vi "simulate (multiple).vi"(2 "liability?  (benefit)":bool, 3 "estimated values":i16[][](array[numeric]), 4 "source data":i16[](array[numeric])) -> (0 "Array":i16[][](array[numeric]), 1 "correct # of elements in source data?":bool)   [LabVIEW 2009]
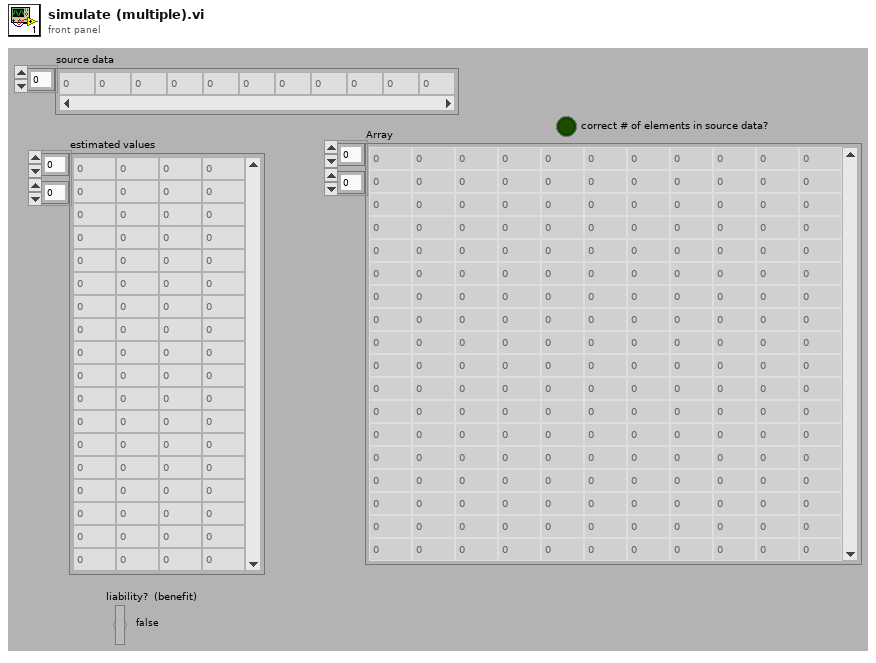
[diagram p1: front panel]
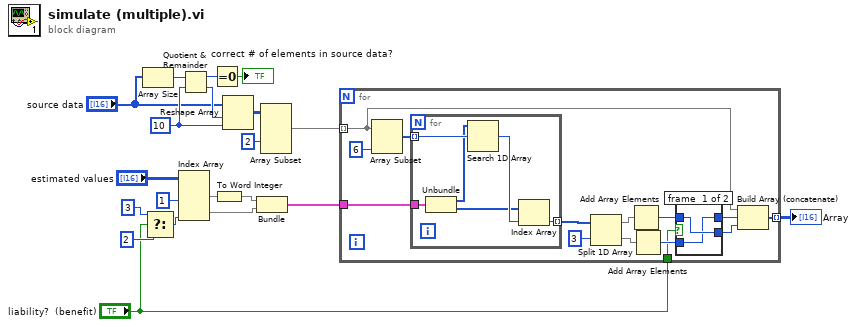
[diagram p0: block diagram]
diagram:
  w16 = 10 ("dimension size")
  n1 = Array Size(array="source data") -> (size(s)=w17:i32)
  n2 = Select(t=3 ("index (col)"), s="liability?  (benefit)", f=2 ("index (col)")) -> (s? t:f=w2:i32)
  n3 = Index Array(array="estimated values", index (col) #1=1 ("disabled index (col)"), index (col) #2=w2) -> (element #1=w19:i16[], element #2=w18:i16[])  [unwired: 2 in]
  n4 = Quotient & Remainder(x=w17, y=w16) -> (x-y*floor(x/y)=w14:i32, floor(x/y)=w15:i32)
  n5 = Equal To 0?(x=w14) -> (x = 0?=→"correct # of elements in source data?":bool)
  n6 = To Word Integer(number=w19) -> (16bit integer=w5:i16[])
  n7 = Reshape Array("source data", w15, w16) -> (w12:i16[][])
  n8 = Bundle(w5, "estimated values"=w18) -> (w9:cluster{i16[], "estimated values":i16[]})  [unwired: 1 in]
  n9 = Array Subset(array=w12, index (col)=2 ("index")) -> (w10:i16[][])  [unwired: 3 in]
  n10 = for {
    tunnel: w10 -> [w26] mode=indexing
    tunnel: w9 -> [w33]
    tunnel: [w27] -> w8 mode=indexing
    tunnel: "liability?  (benefit)" -> [w21]
    n11 = Array Subset(array=w26, length=6) -> (w32:i16[])  [unwired: 1 in]
    n12 = for {
      tunnel: w33 -> [w43]
      tunnel: w32 -> [w44] mode=indexing
      tunnel: [w39] -> w31 mode=indexing
      n13 = Unbundle(w43) -> (w42:i16[], "estimated values"=w40:i16[])
      n14 = Search 1D Array(1D array=w42, element=w44) -> (index of element=w41:i32)  [unwired: 1 in]
      n15 = Index Array(array=w40, index=w41) -> (element=w39:i16)
    }
    n16 = Split 1D Array(array=w31, index=3) -> (first subarray=w29:i16[], second subarray=w28:i16[])
    n17 = Add Array Elements(numeric array=w29) -> (sum=w25:i16)
    n18 = Add Array Elements(numeric array=w28) -> (sum=w23:i16)
    n19 = case shown="True" w21 {
      tunnel: w25 -> [w36 w38]
      tunnel: [w35 w38] -> w24
      tunnel: [w36 w37] -> w22
      tunnel: w23 -> [w35 w37]
      frame #0 {
      }
      frame #1 {
      }
    }
    n20 = Build Array (concatenate)(w26, w24, w22) -> (w27:i16[])
  }
  "Array" <- w8
